vi "example_absorption.vi"() -> ()   [LabVIEW 2015]
panel:
  out "mHT":dbl=0.004070823872413185 format="%#_16g"
  in  "Input Parameters Cluster":T1={"nu0"=112265.5949, "GammaD"=0.0351, "Gamma0"=0.0117, "Gamma2"=0.0054, "Delta0"=0.0305, "Delta2"=0.0124, "NuOptRe"=0.038, "NuOptIm"=-0.0175, "nu"=112266.5949, "Xlm"=0.001, "Ylm"=0.0005, "alpha"=1.98573285442, "disp"=enum."Absorption"} {"alpha" format="%#_16f"; "Ylm" format="%#_16f"; "Xlm" format="%#_16f"; "nu0" format="%#_16g"; "GammaD" format="%#_16f"; "Gamma0" format="%#_16f"; "Gamma2" format="%#_16f"; "Delta0" format="%#_16f"; "Delta2" format="%#_16f"; "NuOptRe" format="%#_16f"; "NuOptIm" format="%#_16f"; "nu" format="%#_16f"}
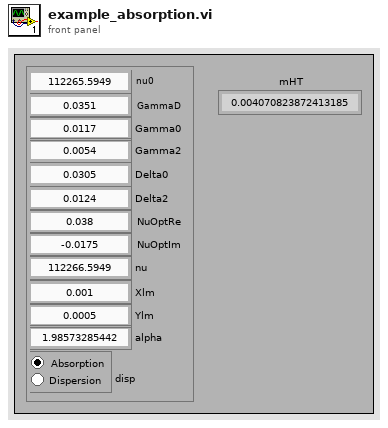
[diagram p1: front panel]
types:
  T1 = cluster{"nu0":dbl, "GammaD":dbl, "Gamma0":dbl, "Gamma2":dbl, "Delta0":dbl, "Delta2":dbl, "NuOptRe":dbl, "NuOptIm":dbl, "nu":dbl, "Xlm":dbl, "Ylm":dbl, "alpha":dbl, "disp":enum32{"Absorption", "Dispersion"}}
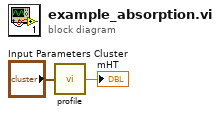
[diagram p0: block diagram]
diagram:
  n1 = call "profile.vi"("Input Parameters Cluster"="Input Parameters Cluster") -> ("mHT"=→"mHT":dbl)
